vi "set_config_cluster.vi"(8 "error in (no error)":errorcluster, 10 "config cluster variant":variant, 11 "DAQmxDigitalOut in":refnum<class "DigitalOutDL110325DAQmx.lvclass">) -> (0 "error out":errorcluster, 3 "DAQmxDigitalOut out":refnum<class "DigitalOutDL110325DAQmx.lvclass">)   [LabVIEW 2010, in "DigitalOutDL110325DAQmx.lvclass"]
uses:
  DigitalOutDL110325DAQmx.lvclass
  DigitalOutDL110325DAQmx.lvclass/DigitalOutDL110325DAQmx.ctl
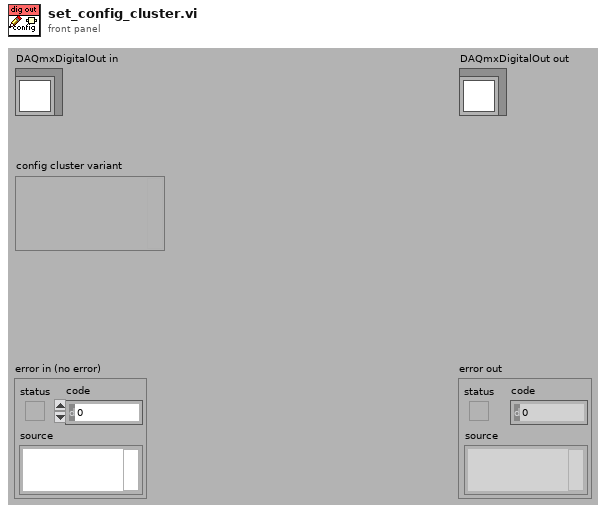
[diagram p1: front panel]
types:
  T1 = typedef "DigitalOutDL110325DAQmx.lvclass/config_data_cluster.ctl" = cluster{"digital output line":string}
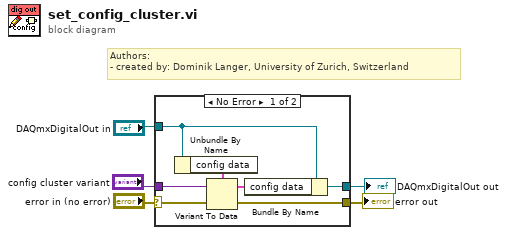
[diagram p0: block diagram]
diagram:
  # "Authors: \n- created by: Dominik Langer, University of Zurich, Switzerland"
  n1 = case shown="No Error" "error in (no error)" {
    selector: "error in (no error)" -> [w10 w13]
    tunnel: "DAQmxDigitalOut in" -> [w8 w14]
    tunnel: [w7 w13] -> w2
    tunnel: [w6 w14] -> w1
    tunnel: "config cluster variant" -> [w9 _]
    frame No Error {
      n2 = Unbundle By Name(w8) -> ("config data"=w12:T1)
      n3 = Variant To Data(error in=w10, Variant=w9, type=w12) -> (error out=w7:errorcluster, data=w11:T1)
      n4 = Bundle By Name(cluster=w8, "config data"=w11) -> (w6:refnum<class "DigitalOutDL110325DAQmx.lvclass">)
    }
    frame Error {
    }
  }
  "error out" <- w2
  "DAQmxDigitalOut out" <- w1
